vi "Get CAN Frame Changes.vi"(8 "error in (no error)":errorcluster, 9 "New Cluster":refnum<k21>, 10 "Database Changes":T1 {"Missing"."Node Ref" format="%.0x"; "Changed"."Old"."Node Ref" format="%.0x"}, 11 "TreeControl in":refnum<vi>) -> (0 "error out":errorcluster, 2 "Change":T8 {"Frames to Delete" format="%.0x"; "Frames to Update"."Node Ref" format="%.0x"}, 3 "TreeControl out":refnum<vi>)   [LabVIEW 2025, in "Protection and Counter Addon System Explorer.lvlib"]
uses:
  Protection and Counter Addon System Explorer.lvlib
  Types/CAN Update Results.ctl
  <vilib>/NI VeriStand/Custom Device API/Custom Device Item Ref.ctl
  Types/CAN Frame Update Results.ctl
  Types/CAN Filter Type.ctl
  Types/Base Frame Info_NoVS.ctl
  Types/Database Changes.ctl
  Types/Base Frame Info.ctl
  Types/Related CAN Frames.ctl
  Types/Related CAN Frames No VS.ctl
  <vilib>/NI VeriStand/Custom Device API/Custom Device API.lvlib
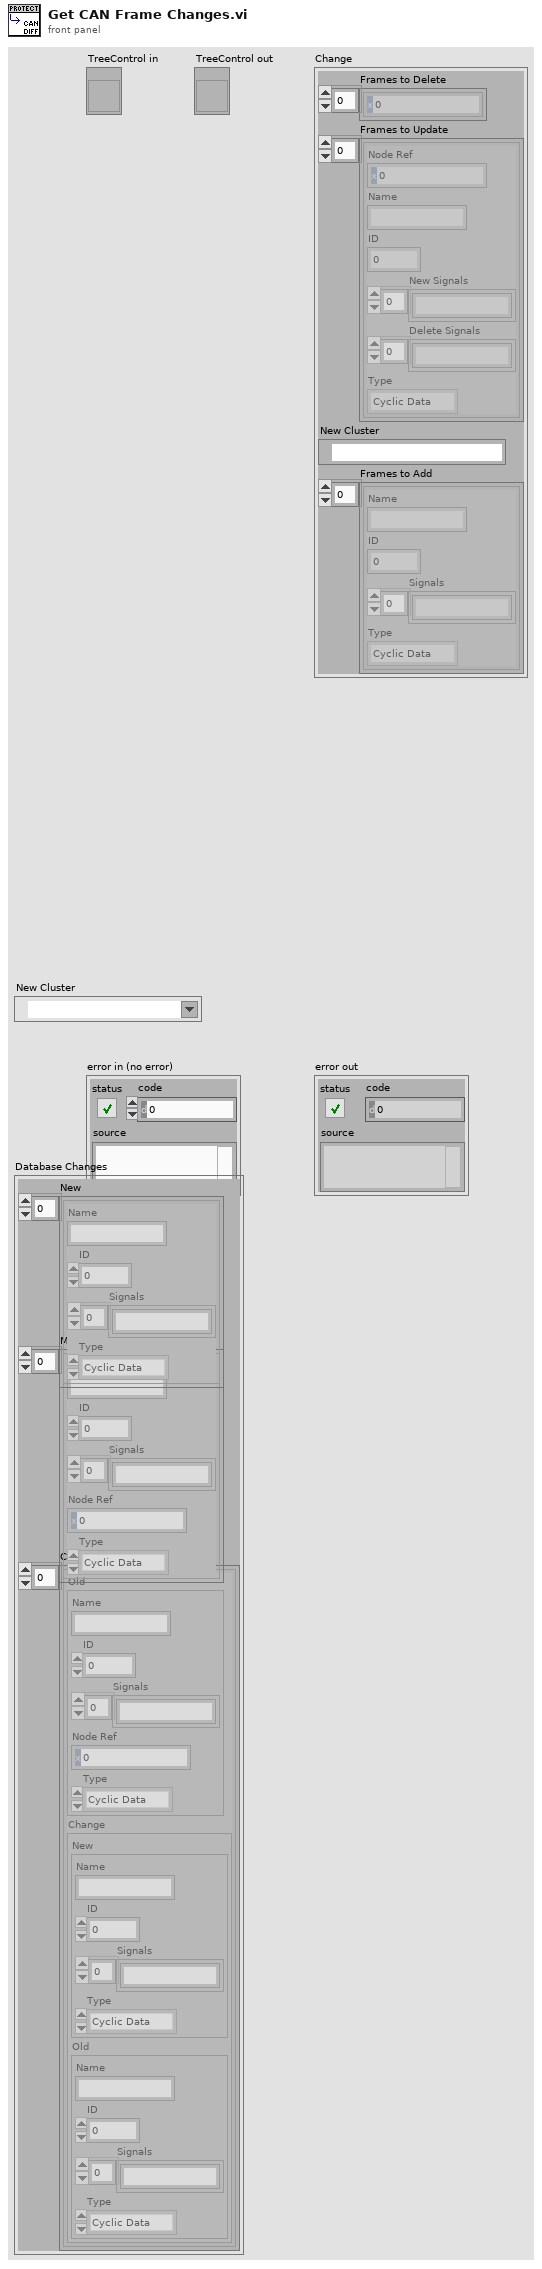
[diagram p1: front panel]
types:
  T1 = typedef "Protection and Counter Addon System Explorer.lvlib/Database Changes.ctl" = cluster{"New":T2[], "Missing":T4[], "Changed":T6[]}
  T2 = typedef "Protection and Counter Addon System Explorer.lvlib/Base Frame Info_NoVS.ctl" = cluster{"Name":string, "ID":u32, "Signals":string[], "Type":T3}
  T3 = typedef "Protection and Counter Addon System Explorer.lvlib/CAN Filter Type.ctl" = enum16{"Cyclic Data", "Event Data", "Cyclic/Event", "All"}
  T4 = typedef "Protection and Counter Addon System Explorer.lvlib/Base Frame Info.ctl" = cluster{"Name":string, "ID":u32, "Signals":string[], "Node Ref":T5, "Type":T3}
  T5 = typedef "Custom Device API.lvlib/Custom Device Item Ref.ctl" = u64
  T6 = typedef "Protection and Counter Addon System Explorer.lvlib/Related CAN Frames.ctl" = cluster{"Old":T4, "Change":T7}
  T7 = typedef "Protection and Counter Addon System Explorer.lvlib/Related CAN Frames No VS.ctl" = cluster{"New":T2, "Old":T2}
  T8 = typedef "Protection and Counter Addon System Explorer.lvlib/CAN Update Results.ctl" = cluster{"Frames to Delete":T5[], "Frames to Update":T9[], "New Cluster":refnum<k21>, "Frames to Add":T2[]}
  T9 = typedef "Protection and Counter Addon System Explorer.lvlib/CAN Frame Update Results.ctl" = cluster{"Node Ref":T5, "Name":string, "ID":u32, "New Signals":string[], "Delete Signals":string[], "Type":T3}
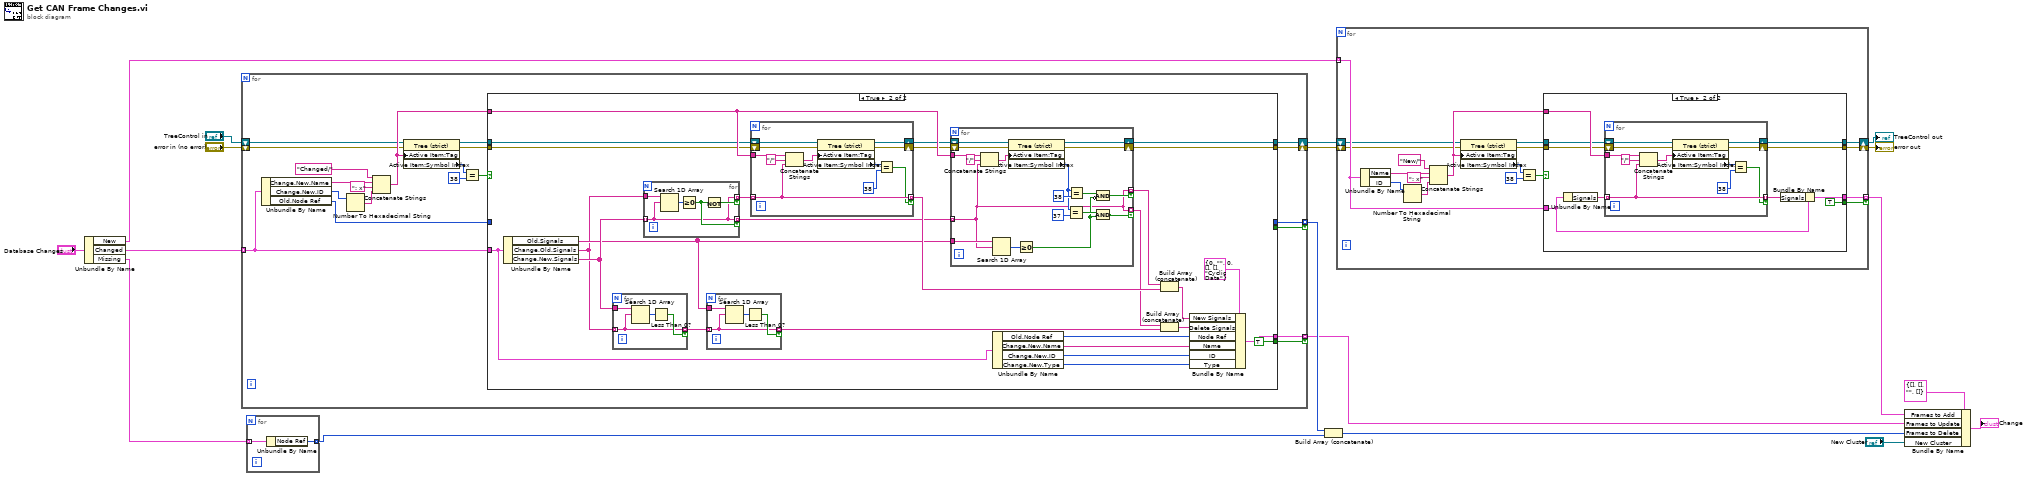
[diagram p0: block diagram]
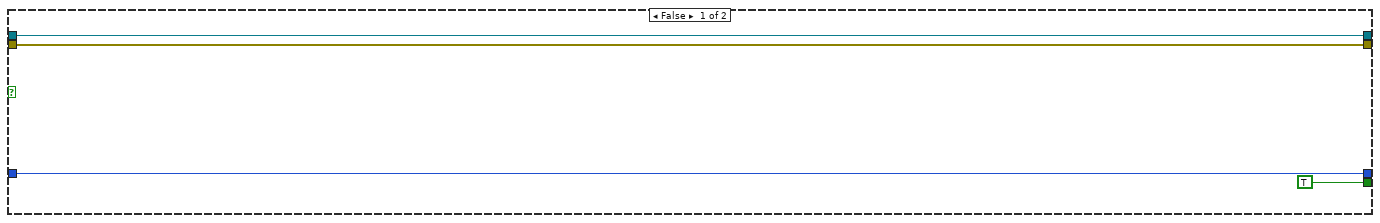
[diagram p2: hidden frame]
diagram:
  n1 = Unbundle By Name("Database Changes") -> ("New"=w7:T2[], "Changed"=w12:T6[], "Missing"=w11:T4[])
  n2 = for {
    tunnel: w12 -> [w32] mode=indexing
    tunnel: [w24] -> w16 mode=indexing if=w23
    tunnel: [w30] -> w8 mode=indexing if=w22
    shift-right: [w20] -> w6
    shift-left: "error in (no error)" -> [w27]
    shift-right: [w21] -> w4
    shift-left: "TreeControl in" -> [w26]
    n3 = Unbundle By Name(w32) -> ("Change.New.Name"=w39:string, "Change.New.ID"=w37:u32, "Old.Node Ref"=w25:T5)
    n4 = Number To Hexadecimal String(2:w37) -> (0:w36:string)  [unwired: 1 in]
    n5 = Concatenate Strings("Changed/" ("string"), w39, ": x" ("string"), w36) -> (w33:string)
    n6 = property class="Tree (strict)"(reference=w26, error in=w27, "Active Item:Tag"=w33) -> (reference out=w31:refnum<vi>, error out=w28:errorcluster, "Active Item:Symbol Index"=w35:i32)
    n7 = Equal?(x=w35, y=38 ("Active Item:Symbol Index")) -> (x = y?=w29:bool)
    n8 = case shown="True" w29 {
      tunnel: w33 -> [_ w66]
      tunnel: w32 -> [_ w47]
      tunnel: w31 -> [w40 w64]
      tunnel: [_ w59] -> w30
      tunnel: w25 -> [w43 _]
      tunnel: w28 -> [w41 w56]
      tunnel: [w43 _] -> w24
      tunnel: [TRUE _] -> w23
      tunnel: [_ TRUE] -> w22
      tunnel: [w40 w46] -> w21
      tunnel: [w41 w45] -> w20
      frame False {
      }
      frame True {
        n9 = Unbundle By Name(w47) -> ("Old.Signals"=w63:string[], "Change.Old.Signals"=w55:string[], "Change.New.Signals"=w70:string[])
        n10 = for {
          tunnel: w70 -> [w107]
          tunnel: w55 -> [w104] mode=indexing
          tunnel: [w104] -> w65 mode=indexing if=w105
          n11 = Search 1D Array(1D array=w107, element=w104) -> (index of element=w106:i32)  [unwired: 1 in]
          n12 = Less Than 0?(x=w106) -> (x < 0?=w105:bool)
        }
        n13 = for {
          tunnel: w55 -> [w112]
          tunnel: w70 -> [w108] mode=indexing
          tunnel: [w108] -> w67 mode=indexing if=w110
          tunnel: [w108] -> w69 mode=indexing if=w109
          n14 = Search 1D Array(1D array=w112, element=w108) -> (index of element=w111:i32)  [unwired: 1 in]
          n15 = Greater Or Equal To 0?(x=w111) -> (x >= 0?=w110:bool)
          n16 = Not(x=w110) -> (.not. x?=w109:bool)
        }
        n17 = for {
          tunnel: w63 -> [w74]
          tunnel: w65 -> [w71] mode=indexing
          tunnel: [w71] -> w60 mode=indexing if=w72
          n18 = Search 1D Array(1D array=w74, element=w71) -> (index of element=w73:i32)  [unwired: 1 in]
          n19 = Less Than 0?(x=w73) -> (x < 0?=w72:bool)
        }
        n20 = for {
          tunnel: w66 -> [w101]
          tunnel: w69 -> [w99] mode=indexing
          tunnel: [w99] -> w68 mode=indexing if=w98
          shift-right: [w95] -> w58
          shift-left: w64 -> [w97]
          shift-right: [w94] -> w57
          shift-left: w56 -> [w93]
          n21 = Concatenate Strings(w101, "/" ("string"), w99) -> (w96:string)
          n22 = property class="Tree (strict)"(reference=w97, error in=w93, "Active Item:Tag"=w96) -> (reference out=w95:refnum<vi>, error out=w94:errorcluster, "Active Item:Symbol Index"=w102:i32)
          n23 = Equal?(x=w102, y=38 ("Active Item:Symbol Index")) -> (x = y?=w98:bool)
        }
        n24 = for {
          tunnel: w66 -> [w91]
          tunnel: w67 -> [w80] mode=indexing
          tunnel: [w80] -> w62 mode=indexing if=w83
          tunnel: w63 -> [w85]
          tunnel: [w80] -> w61 mode=indexing if=w79
          shift-right: [w77] -> w46
          shift-left: w58 -> [w78]
          shift-right: [w75] -> w45
          shift-left: w57 -> [w76]
          n25 = Concatenate Strings(w91, "/" ("string"), w80) -> (w89:string)
          n26 = Search 1D Array(1D array=w85, element=w80) -> (index of element=w84:i32)  [unwired: 1 in]
          n27 = property class="Tree (strict)"(reference=w78, error in=w76, "Active Item:Tag"=w89) -> (reference out=w77:refnum<vi>, error out=w75:errorcluster, "Active Item:Symbol Index"=w87:i32)
          n28 = Greater Or Equal To 0?(x=w84) -> (x >= 0?=w81:bool)
          n29 = Equal?(x=w87, y=37 ("Active Item:Symbol Index")) -> (x = y?=w82:bool)
          n30 = Equal?(x=w87, y=38 ("Active Item:Symbol Index")) -> (x = y?=w86:bool)
          n31 = Compound Arithmetic op=AND(w86, invert w81) -> (w83:bool)
          n32 = Compound Arithmetic op=AND(w82, w81) -> (w79:bool)
        }
        n33 = Unbundle By Name(w47) -> ("Old.Node Ref"=w51:T5, "Change.New.Name"=w54:string, "Change.New.ID"=w50:u32, "Change.New.Type"=w44:T3)
        n34 = Build Array (concatenate)(w62, w68) -> (w49:string[])
        n35 = Build Array (concatenate)(w61, w60) -> (w48:string[])
        n36 = Bundle By Name(cluster=T9 {"Node Ref"=0, "Name"="", "ID"=0, "New Signals"=[], "Delete Signals"=[], "Type"=enum."Cyclic Data"}, "New Signals"=w49, "Delete Signals"=w48, "Node Ref"=w51, "Name"=w54, "ID"=w50, "Type"=w44) -> (w59:T9)
      }
    }
  }
  n37 = for {
    tunnel: w11 -> [w114] mode=indexing
    tunnel: [w113] -> w9 mode=indexing
    n38 = Unbundle By Name(w114) -> ("Node Ref"=w113:T5)
  }
  n39 = Build Array (concatenate)(w16, w9) -> (w10:T5[])
  n40 = for {
    tunnel: w7 -> [w125] mode=indexing
    tunnel: [w123] -> w2 mode=indexing if=w118
    shift-right: [w116] -> w5
    shift-left: w6 -> [w120]
    shift-right: [w117] -> w3
    shift-left: w4 -> [w119]
    n41 = Unbundle By Name(w125) -> ("Name"=w132:string, "ID"=w130:u32)
    n42 = Number To Hexadecimal String(2:w130) -> (0:w129:string)  [unwired: 1 in]
    n43 = Concatenate Strings("New/" ("string"), w132, ": x" ("string"), w129) -> (w126:string)
    n44 = property class="Tree (strict)"(reference=w119, error in=w120, "Active Item:Tag"=w126) -> (reference out=w124:refnum<vi>, error out=w121:errorcluster, "Active Item:Symbol Index"=w128:i32)
    n45 = Equal?(x=w128, y=38 ("Active Item:Symbol Index")) -> (x = y?=w122:bool)
    n46 = case shown="True" w122 {
      tunnel: w126 -> [_ w144]
      tunnel: w125 -> [_ w136]
      tunnel: w124 -> [w133 w143]
      tunnel: [_ w142] -> w123
      tunnel: w121 -> [w134 w141]
      tunnel: [_ TRUE] -> w118
      tunnel: [w133 w137] -> w117
      tunnel: [w134 w138] -> w116
      frame False {
      }
      frame True {
        n47 = Unbundle By Name(w136) -> ("Signals"=w139:string[])
        n48 = for {
          tunnel: w144 -> [w153]
          tunnel: w139 -> [w151] mode=indexing
          tunnel: [w151] -> w135 mode=indexing if=w150
          shift-right: [w147] -> w137
          shift-left: w143 -> [w149]
          shift-right: [w146] -> w138
          shift-left: w141 -> [w145]
          n49 = Concatenate Strings(w153, "/" ("string"), w151) -> (w148:string)
          n50 = property class="Tree (strict)"(reference=w149, error in=w145, "Active Item:Tag"=w148) -> (reference out=w147:refnum<vi>, error out=w146:errorcluster, "Active Item:Symbol Index"=w154:i32)
          n51 = Equal?(x=w154, y=38 ("Active Item:Symbol Index")) -> (x = y?=w150:bool)
        }
        n52 = Bundle By Name(cluster=w136, "Signals"=w135) -> (w142:T2)
      }
    }
  }
  "error out" <- w5
  "TreeControl out" <- w3
  n53 = Bundle By Name(cluster=T8 {"Frames to Delete"=[], "Frames to Update"=[], "New Cluster"="", "Frames to Add"=[]}, "Frames to Add"=w2, "Frames to Update"=w8, "Frames to Delete"=w10, "New Cluster"="New Cluster") -> (→"Change":T8)
